vi "parse generic data with strings.vi"(8 "error in":errorcluster, 9 "dataSourceRid":string, 10 "Time Stamp (now: system time)":timestamp format="%<%x %.3X>T", 11 "Data Cluster":variant caption="Data Clusters must only contain scalar values (integers, floats, booleans, or strings). Nested clusters are allowed.") -> (0 "error out":errorcluster, 3 "JSON":string)   [LabVIEW 2020]
uses:
  ed5590e3-c1f7-48d3-8ff7-d9ee3b767263.vi
  a5b7f845-be68-4c9a-ad6c-83d99c3db13b.vi
  88aeaf81-e89a-43ae-9e76-8fa1d67f37f9.vi
  cfe8da2e-4b12-4f12-b932-2a0625bc18f4.vi
  4609e594-e62c-4725-984f-cc1e22b184a7.vi
  01dc9cd7-1da2-47da-a8d7-1150ed450fbb.vi
  1a77bec5-1a35-43cc-b640-5a18640e21d6.vi
  b5184ad7-a107-4c31-b670-5c4db2b6eaac.vi
  d7255a6e-ae9a-40df-94e1-f7199c397288.vi
  5171cadf-4f01-4683-b61d-c49ebc1a03d1.vi
  bd4dc24f-41f2-4310-95cd-0bf77e7af417.vi
  <vilib>/LabVIEW Open Source Project/Epoch Date & Time/epoch.UNIX/Epoch.UNIX.lvclass
  C:/Program Files/National Instruments/LabVIEW 2020/vi.lib/LabVIEW Open Source Project/Epoch Date & Time/epoch/Epoch.lvclass
  <vilib>/LabVIEW Open Source Project/Epoch Date & Time/Get Epoch Time.vi
  <vilib>/JDP Science/JSONtext/Variant to JSON Text.vi
  <vilib>/JDP Science/JSONtext/support/Format JSON Array Text.vi
  <vilib>/JDP Science/JSONtext/LVClass Serializer/JSONtext LVClass Serializer.lvclass
  <userlib>/_OpenG.lib/lvdata/lvdata.llb/openg_variant.lvlib
  <vilib>/JDP Science/JSONtext/JSONtext.lvlib
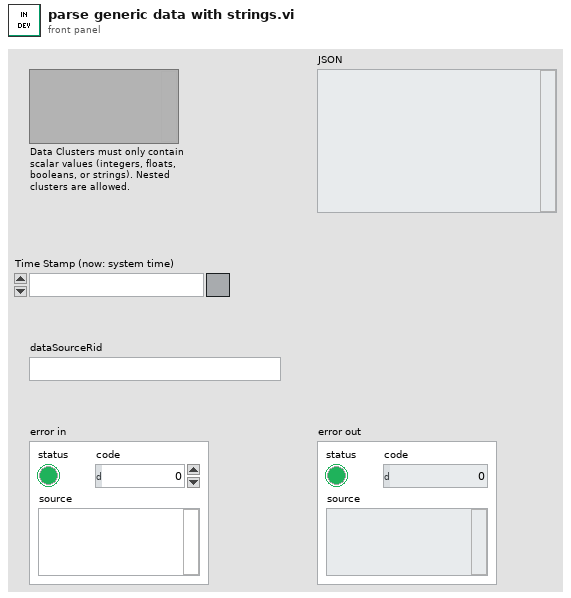
[diagram p1: front panel]
types:
  T1 = typedef "openg_variant.lvlib/Type Descriptor Enumeration__ogtk.ctl" = enum8{"<Null>", "I8", "I16", "I32", "I64", "U8", "U16", "U32", "U64", "SGL", "DBL", "EXT", "CSG", "CDB", "CXT", "0x0F", "0x10", "0x11", "0x12", "0x13", "0x14", "Enum U8", "Enum U16", "Enum U32", "Enum U64", "SGL PQ", "DBL PQ", "EXT PQ", "CSG PQ", "CDB PQ", "CXT PQ", "0x1F", "0x20", "Boolean", "0x22", "0x23", "0x24", "0x25", "0x26", "0x27", "0x28", "0x29", "0x2A", "0x2B", "0x2C", "0x2D", "0x2E", "0x2F", "String", "0x31", "Path", "Pict", "0x34", "0x35", "0x36", "DAQ", "0x38", "0x39", "0x3A", "0x3B", "0x3C", "0x3D", "0x3E", "0x3F", "Array", "0x41", "0x42", "0x43", "0x44", "0x45", "0x46", "0x47", "0x48", "0x49", "0x4A", "0x4B", "0x4C", "0x4D", "0x4E", "0x4F", "Cluster", "0x51", "0x52", "Variant", "Waveform", "0x55", "0x56", "0x57", "0x58", "0x59", "0x5A", "0x5B", "0x5C", "0x5D", "0x5E", "Fixed Point", "0x60", "0x61", "0x62", "0x63", "0x64", "0x65", "0x66", "0x67", "0x68", "0x69", "0x6A", "0x6B", "0x6C", "0x6D", "0x6E", "0x6F", "Refnum", "0x71", "0x72", "Set Collection", "Map Collection"}
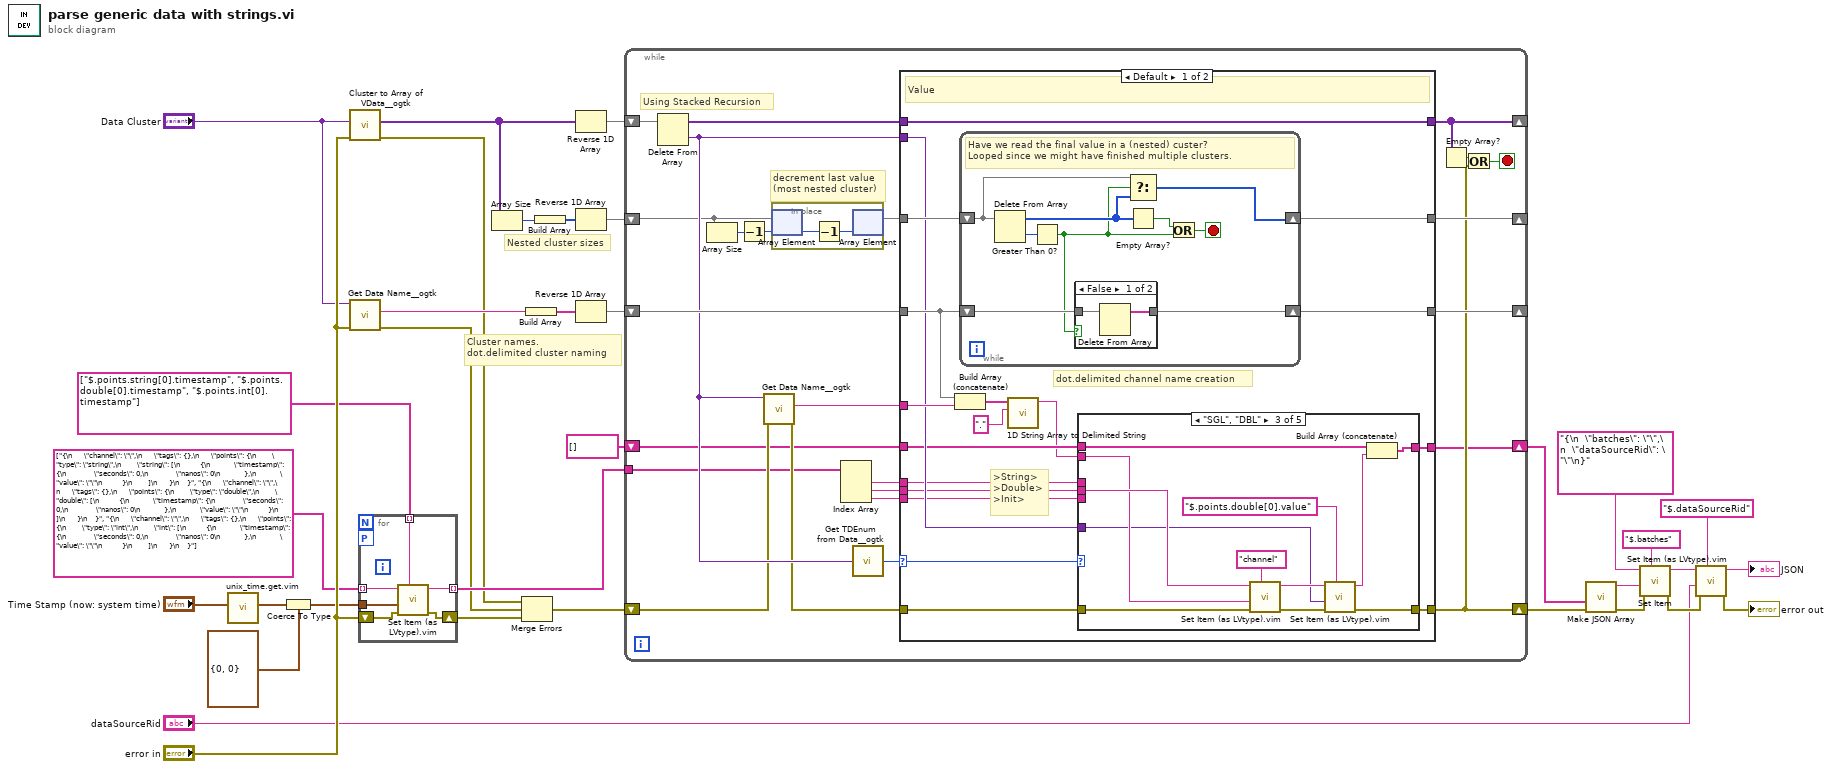
[diagram p0: block diagram]
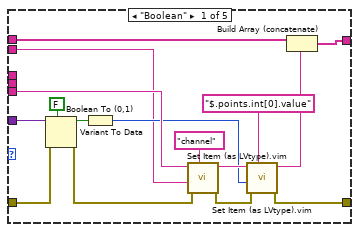
[diagram p2: hidden frame]
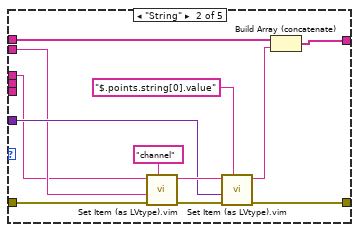
[diagram p3: hidden frame]
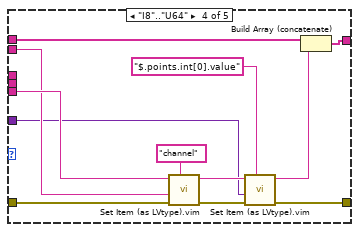
[diagram p4: hidden frame]
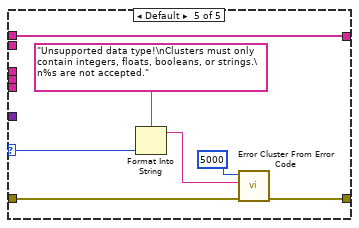
[diagram p5: hidden frame]
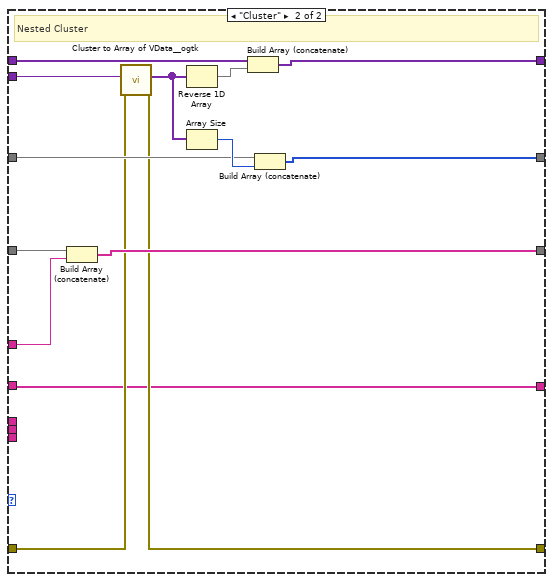
[diagram p7: hidden frame]
diagram:
  # "Nested cluster sizes"
  # "Cluster names.\ndot.delimited cluster naming"
  n1 = call "unix_time.get.vim"("Time Stamp (empty: now) [single or array]"="Time Stamp (now: system time)") -> ("UNIX Timestamp"=w24:cluster{"Seconds":i64, "Nanoseconds":i64})  [unwired: 10 in]
  n2 = Coerce To Type(0:w24, 1:cluster{"seconds":i32, "nanos":i32} {"seconds"=0, "nanos"=0} ("UNIX Timestamp")) -> (2:w23:cluster{"seconds":i32, "nanos":i32})
  n3 = call <userlib>:"Cluster to Array of VData__ogtk.vi"("error in (no error)"="error in", "Cluster"="Data Cluster") -> ("error out"=w9:errorcluster, "Array of VData"=w33:variant[])  [unwired: 8 in]
  n4 = call <userlib>:"Get Data Name__ogtk.vi"("error in (no error)"="error in", "Data"="Data Cluster") -> ("error out"=w8:errorcluster, "Data Name"=w32:string)  [unwired: 7 in, 1 out]
  n5 = for {
    tunnel: w23 -> [w40]
    tunnel: [w39] -> w22 mode=indexing
    tunnel: string[] ["{\n      \"channel\": \"\",\n      \"tags\": {},\n      \"points\": {\n        \"type\": \"string\",\n        \"string\": [\n          {\n            \"timestamp\": {\n              \"seconds\": 0,\n              \"nanos\": 0\n            },\n            \"value\": \"\"\n          }\n        ]\n      }\n    }", "{\n      \"channel\": \"\",\n      \"tags\": {},\n      \"points\": {\n        \"type\": \"double\",\n        \"double\": [\n          {\n            \"timestamp\": {\n              \"seconds\": 0,\n              \"nanos\": 0\n            },\n            \"value\": \"\"\n          }\n        ]\n      }\n    }", "{\n      \"channel\": \"\",\n      \"tags\": {},\n      \"points\": {\n        \"type\": \"int\",\n        \"int\": [\n          {\n            \"timestamp\": {\n              \"seconds\": 0,\n              \"nanos\": 0\n            },\n            \"value\": \"\"\n          }\n        ]\n      }\n    }"] -> [w38] mode=indexing
    tunnel: string[] ["$.points.string[0].timestamp", "$.points.double[0].timestamp", "$.points.int[0].timestamp"] -> [w37] mode=indexing
    shift-right: [w35] -> w4
    shift-left: "error in" -> [w36]
    workers-P: _ -> [_]
    n6 = call "Set Item (as LVtype).vim"("$Path or Item Name"=w37, "error in (no error)"=w36, "Anything"=w40, "JSON"=w38) -> ("error out"=w35:errorcluster, "<JSON>"=w39:string)  [unwired: 4 in, 1 out]
  }
  n7 = Array Size(array=w33) -> (size(s)=w31:i32)
  n8 = Merge Errors(w9, w8, w4) -> (w7:errorcluster)
  n9 = Build Array(w32) -> (w29:string[])
  n10 = Build Array(w31) -> (w30:i32[])
  n11 = Reverse 1D Array(array=w33) -> (reversed array=w28:variant[])
  n12 = Reverse 1D Array(array=w30) -> (reversed array=w27:i32[])
  n13 = Reverse 1D Array(array=w29) -> (reversed array=w26:string[])
  n14 = while {
    shift-right: [w59] -> _
    shift-left: w28 -> [w64]
    shift-right: [w61] -> _
    shift-left: w26 -> [w60]
    shift-right: [w58] -> _
    shift-left: w27 -> [w44]
    shift-right: [w55] -> w12
    shift-left: w7 -> [w52]
    tunnel: w22 -> [w45]
    shift-right: [w50] -> w20
    shift-left: string[] [] ("<JSON>") -> [w49]
    stop <- w56 stop-if-true
    # "Using Stacked Recursion"
    # "decrement last value\n(most nested cluster)"
    n15 = Delete From Array(array=w64) -> (deleted portion=w54:variant, array with subset deleted=w62:variant[])  [unwired: 2 in]
    n16 = Array Size(array=w44) -> (size(s)=w42:i32)
    n17 = Decrement(x=w42) -> (x-1=w41:i32)
    n18 = call <userlib>:"Get Data Name__ogtk.vi"("error in (no error)"=w52, "Data"=w54) -> ("error out"=w51:errorcluster, "Data Name"=w53:string)  [unwired: 7 in, 1 out]
    n19 = in-place {
      n20 = in-place-array #1(w44, w41) -> (w66:i32)
      n21 = Decrement(x=w66) -> (x-1=w65:i32)
      n22 = in-place-array #1(w65) -> (w43:i32[])  [unwired: 1 out]
    }
    n23 = Index Array(array=w45) -> (element #1=w46:string, element #2=w47:string, element #3=w48:string)  [unwired: 3 in]
    n24 = call <userlib>:"Get TDEnum from Data__ogtk.vi"("Data"=w54) -> ("Type Descriptor Enumeration"=w63:T1)  [unwired: 4 in]
    n25 = case shown="Default" w63 {
      selector: w63 -> [w76 _]
      tunnel: w54 -> [w75 w160]
      tunnel: [w84 w167] -> w59
      tunnel: w62 -> [w84 w168]
      tunnel: [w80 w161] -> w61
      tunnel: w60 -> [w79 w166]
      tunnel: w53 -> [w78 w165]
      tunnel: [w81 w163] -> w58
      tunnel: w43 -> [w82 w162]
      tunnel: w51 -> [w74 w159]
      tunnel: [w73 w158] -> w55
      tunnel: w46 -> [w72 _]
      tunnel: w47 -> [w71 _]
      tunnel: w48 -> [w70 _]
      tunnel: [w69 w156] -> w50
      tunnel: w49 -> [w68 w156]
      frame Default {
        # "dot.delimited channel name creation"
        # ">String>\n>Double>\n>Init>"
        # "Value"
        n26 = Build Array (concatenate)(w79, w78) -> (w77:string[])
        n27 = while {
          shift-right: [w151] -> w81
          shift-left: w82 -> [w152]
          shift-right: [w145] -> w80
          shift-left: w79 -> [w147]
          stop <- w148 stop-if-true
          # "Have we read the final value in a (nested) custer?\nLooped since we might have finished multiple clusters."
          n28 = Delete From Array(array=w152) -> (deleted portion=w144:i32, array with subset deleted=w150:i32[])  [unwired: 2 in]
          n29 = Greater Than 0?(x=w144) -> (x > 0?=w146:bool)
          n30 = case shown="False" w146 {
            tunnel: w147 -> [w154 w155]
            tunnel: [w153 w155] -> w145
            frame False {
              n31 = Delete From Array(array=w154) -> (array with subset deleted=w153:string[])  [unwired: 2 in, 1 out]
            }
            frame True {
            }
          }
          n32 = Select(t=w152, s=w146, f=w150) -> (s? t:f=w151:i32[])
          n33 = Empty Array?(array=w150) -> (empty?=w149:bool)
          n34 = Or(x=w149, y=w146) -> (x .or. y?=w148:bool)
        }
        n35 = call <vilib>:"1D String Array to Delimited String.vi"("delimiter"=".", "string array"=w77) -> ("delimited string"=w67:string)  [unwired: 9 in]
        n36 = case shown="\"SGL\", \"DBL\"" w76 {
          selector: w76 -> [_ _ _ _ w142]
          tunnel: w75 -> [w100 w109 w118 w126 _]
          tunnel: w74 -> [w97 w104 w119 w125 w139]
          tunnel: [w90 w105 w116 w130 w138] -> w73
          tunnel: w72 -> [_ w107 _ _ _]
          tunnel: w71 -> [_ _ w121 _ _]
          tunnel: w70 -> [w93 _ _ w135 _]
          tunnel: w67 -> [w88 w108 w120 w134 _]
          tunnel: [w86 w101 w113 w127 w137] -> w69
          tunnel: w68 -> [w87 w103 w115 w129 w137]
          frame "Boolean" {
            n37 = Variant To Data(error in=w97, type=FALSE, Variant=w100) -> (data=w98:bool, error out=w92:errorcluster)
            n38 = Boolean To (0,1)(Boolean=w98) -> (0, 1=w89:i16)
            n39 = call "Set Item (as LVtype).vim"("$Path or Item Name"="channel" ("Name"), "error in (no error)"=w92, "Anything"=w88, "JSON"=w93) -> ("error out"=w91:errorcluster, "<JSON>"=w94:string)  [unwired: 4 in, 1 out]
            n40 = call "Set Item (as LVtype).vim"("$Path or Item Name"="$.points.int[0].value" ("Name"), "error in (no error)"=w91, "Anything"=w89, "JSON"=w94) -> ("error out"=w90:errorcluster, "<JSON>"=w85:string)  [unwired: 4 in, 1 out]
            n41 = Build Array (concatenate)(w87, w85) -> (w86:string[])
          }
          frame "String" {
            n42 = call "Set Item (as LVtype).vim"("$Path or Item Name"="channel" ("Name"), "error in (no error)"=w104, "Anything"=w108, "JSON"=w107) -> ("error out"=w106:errorcluster, "<JSON>"=w110:string)  [unwired: 4 in, 1 out]
            n43 = call "Set Item (as LVtype).vim"("$Path or Item Name"="$.points.string[0].value" ("Name"), "error in (no error)"=w106, "Anything"=w109, "JSON"=w110) -> ("error out"=w105:errorcluster, "<JSON>"=w102:string)  [unwired: 4 in, 1 out]
            n44 = Build Array (concatenate)(w103, w102) -> (w101:string[])
          }
          frame "SGL", "DBL" {
            n45 = call "Set Item (as LVtype).vim"("$Path or Item Name"="channel" ("Name"), "error in (no error)"=w119, "Anything"=w120, "JSON"=w121) -> ("error out"=w117:errorcluster, "<JSON>"=w122:string)  [unwired: 4 in, 1 out]
            n46 = call "Set Item (as LVtype).vim"("$Path or Item Name"="$.points.double[0].value" ("Name"), "error in (no error)"=w117, "Anything"=w118, "JSON"=w122) -> ("error out"=w116:errorcluster, "<JSON>"=w114:string)  [unwired: 4 in, 1 out]
            n47 = Build Array (concatenate)(w115, w114) -> (w113:string[])
          }
          frame "I8".."U64" {
            n48 = call "Set Item (as LVtype).vim"("$Path or Item Name"="channel" ("Name"), "error in (no error)"=w125, "Anything"=w134, "JSON"=w135) -> ("error out"=w131:errorcluster, "<JSON>"=w132:string)  [unwired: 4 in, 1 out]
            n49 = call "Set Item (as LVtype).vim"("$Path or Item Name"="$.points.int[0].value" ("Name"), "error in (no error)"=w131, "Anything"=w126, "JSON"=w132) -> ("error out"=w130:errorcluster, "<JSON>"=w128:string)  [unwired: 4 in, 1 out]
            n50 = Build Array (concatenate)(w129, w128) -> (w127:string[])
          }
          frame Default {
            n51 = Format Into String(format string="Unsupported data type!\nClusters must only contain integers, floats, booleans, or strings.\n%s are not accepted." ("message"), w142) -> (resulting string=w140:string)  [unwired: 2 in, 1 out]
            n52 = call <vilib>:"Error Cluster From Error Code.vi"("error in (no error)"=w139, "error message (\"\")"=w140, "error code (0)"=5000) -> ("error out"=w138:errorcluster)  [unwired: 6 in]
          }
        }
      }
      frame "Cluster" {
        # "Nested Cluster"
        n53 = Build Array (concatenate)(w166, w165) -> (w161:string[])
        n54 = call <userlib>:"Cluster to Array of VData__ogtk.vi"("error in (no error)"=w159, "Cluster"=w160) -> ("error out"=w158:errorcluster, "Array of VData"=w157:variant[])  [unwired: 8 in]
        n55 = Reverse 1D Array(array=w157) -> (reversed array=w169:variant[])
        n56 = Array Size(array=w157) -> (size(s)=w164:i32)
        n57 = Build Array (concatenate)(w168, w169) -> (w167:variant[])
        n58 = Build Array (concatenate)(w162, w164) -> (w163:i32[])
      }
    }
    n59 = Empty Array?(array=w59) -> (empty?=w57:bool)
    n60 = Or(x=w57, y=w55) -> (x .or. y?=w56:bool)
  }
  n61 = call <vilib>:"Make JSON Array.vi"("error in (no error)"=w12, "JSON Elements"=w20) -> ("error out"=w13:errorcluster, "<JSON>"=w18:string)  [unwired: 8 in]
  n62 = call <vilib>:"Set Item.vi"("$Path or Item Name"="$.batches", "error in (no error)"=w13, "JSON to Insert"=w18, "JSON"="{\n  \"batches\": \"\",\n  \"dataSourceRid\": \"\"\n}") -> ("error out"=w14:errorcluster, "<JSON>"=w15:string)  [unwired: 4 in, 1 out]
  n63 = call "Set Item (as LVtype).vim"("$Path or Item Name"="$.dataSourceRid", "error in (no error)"=w14, "Anything"="dataSourceRid", "JSON"=w15) -> ("error out"=→"error out":errorcluster, "<JSON>"=→"JSON":string)  [unwired: 4 in, 1 out]
